vi "Write File.vi"(8 "error in (no error)":errorcluster, 11 "Data in":refnum<class "Data.lvclass">) -> (0 "error out":errorcluster, 3 "Data out":refnum<class "Data.lvclass">)   [LabVIEW 2016, in "Data.lvclass"]
uses:
  Data.lvclass
  Data.lvclass/Data.ctl
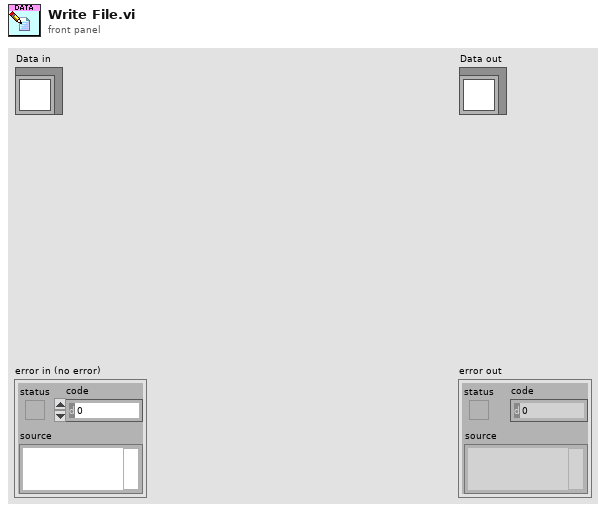
[diagram p1: front panel]
types:
  T1 = typedef "Data.lvclass/Type--enum.ctl" = enum16{"DAT", "ITX", "HDF5", "TDMS", "VI"}
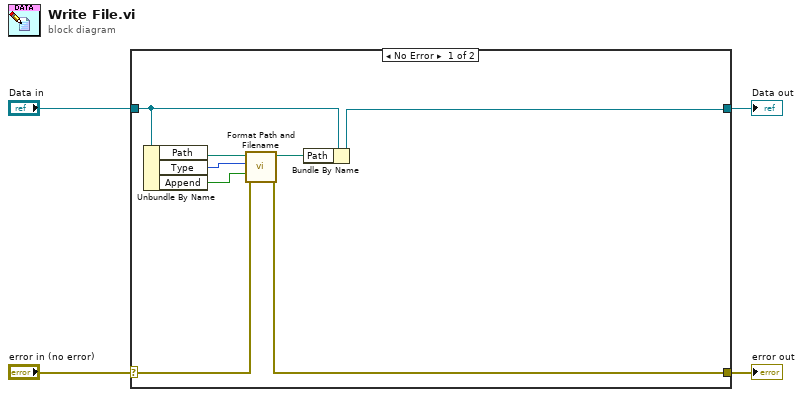
[diagram p0: block diagram]
diagram:
  n1 = case shown="No Error" "error in (no error)" {
    selector: "error in (no error)" -> [w7 w14]
    tunnel: [w9 w14] -> w3
    tunnel: [w10 w13] -> w1
    tunnel: "Data in" -> [w8 w13]
    frame No Error {
      n2 = Unbundle By Name(w8) -> ("Path"=w12:path, "Type"=w5:T1, "Append"=w6:bool)
      n3 = call "Format Path and Filename.vi"("error in"=w7, "append? (F)"=w6, "Type (TDMS)"=w5, "path"=w12) -> ("error out"=w9:errorcluster, "path"=w11:path)  [unwired: 5 in, 1 out]
      n4 = Bundle By Name(cluster=w8, "Path"=w11) -> (w10:refnum<class "Data.lvclass">)
    }
    frame Error {
    }
  }
  "error out" <- w3
  "Data out" <- w1
